vi "osa_main.vi"() -> ()   [LabVIEW 2021]
uses:
  <vilib>/Instr/_visa.llb/Select Event Type.ctl
  osa_globals.vi
  <vilib>/Instr/_visa.llb/VISA Configure Serial Port (Instr).vi
  <vilib>/ErrorRing/Error Ring.xnode
panel:
  in  "apply changes":bool
  in  "OSB status/sensor control":i32(listbox)
  in  "serial timeout (ms)":u32=15000
  out "busy...":bool
  out "LUT":variant
  out "data file refnum":refnum<file>
  in  "teensy port":refnum<visa-resource-name>[](array[refnum])
  out "reset result":bool[](array[boolean])
  out "test result":bool[](array[boolean])
  out "teensy mounted":bool[](array[boolean])
  out "display":T1
  out "elapsed time":string="00:00:00.000"
  out "start time":timestamp format="%<%H:%M:%S%3u>T"
  in  "sensor map settings":cluster{"OSB index":u8[], "display index":i32[]}={"OSB index"=[1, 2, 3, 4, 5, 6, 7], "display index"=[26, 22, 18, 14, 10, 6, 2]}
  in  "save data":bool
  in  "data folder":path
  out "OSA status":string
  out "measuring...":bool
  in  "precision (Hz)":dbl=0.1
  in  "HS frequency (Hz)":dbl=0.5
  in  "OS frequency (Hz)":dbl=1.0
  in  "stop measurement":bool
  in  "start measurement":bool
  in  "reset":bool
  in  "test":bool
  in  "init":bool
  in  "stop VI":bool
  in  "OSB mounted":i32[](listbox)
  # "odor sensor array: main panel"
  # "Each OSB occupies 4 pixels in width on the display screens; set the display index to be which pixel you want the mid-point of the OSB short edge to be located within; no need to touch this unless doing free POGO-pin mounting"
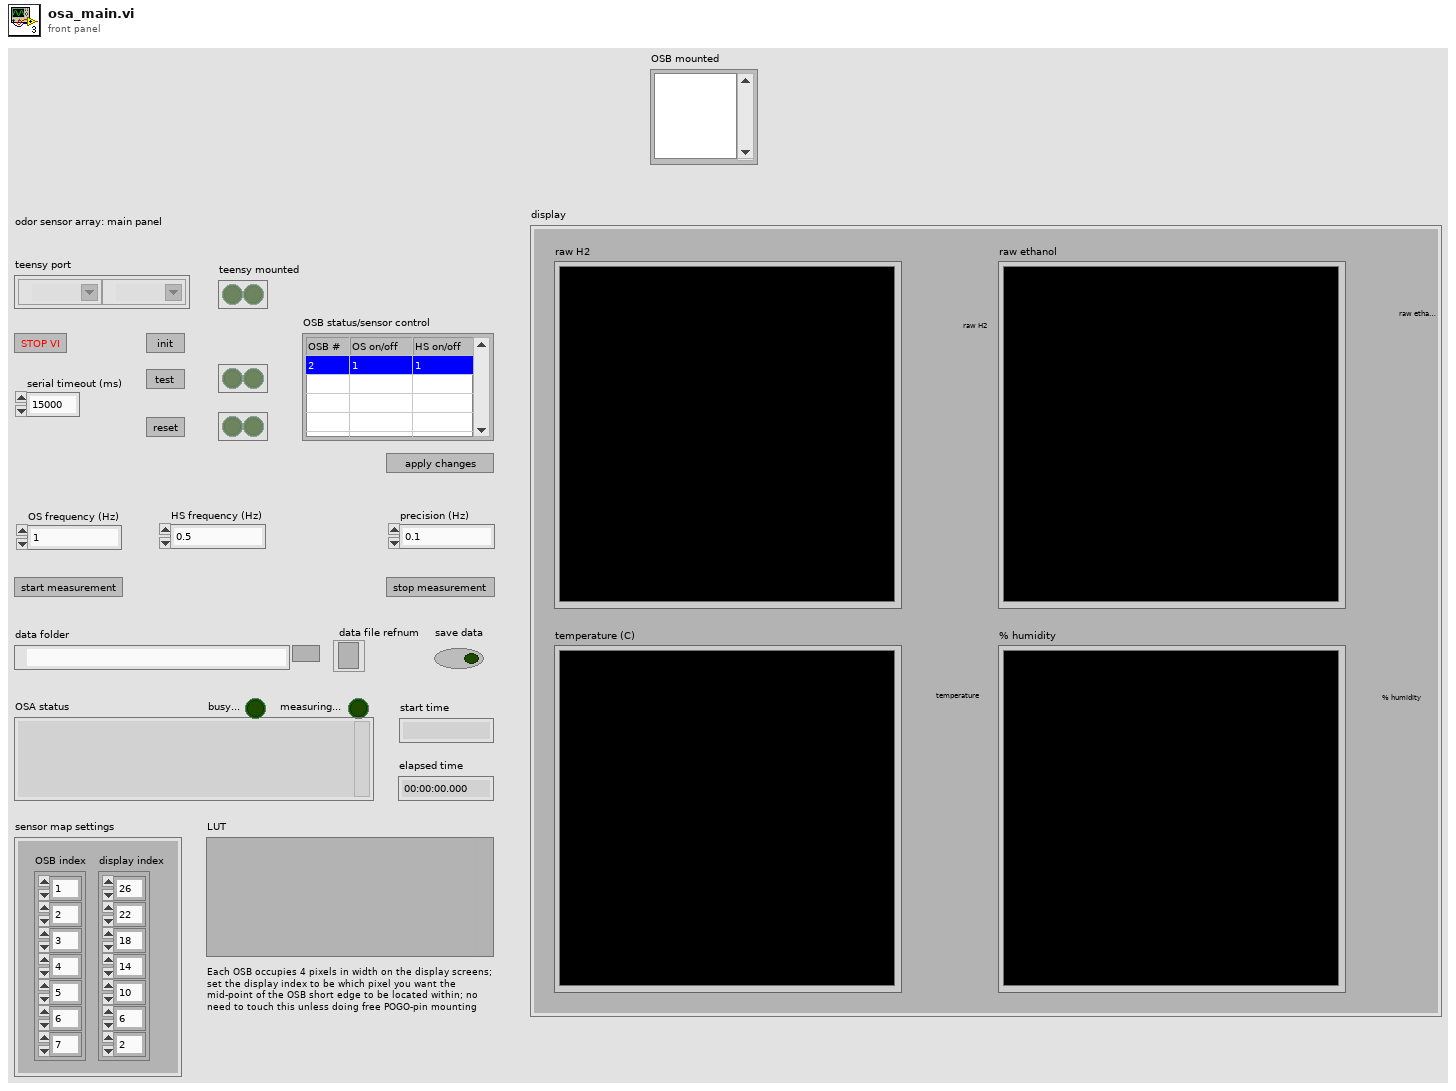
[diagram p1: front panel]
types:
  T1 = cluster{"raw ethanol":dbl[][], "raw H2":dbl[][], "temperature (C)":dbl[][], "% humidity":dbl[][]}
  T2 = cluster{"raw H2":refnum<vi>, "raw ethanol":refnum<vi>, "temperature (C)":refnum<vi>, "% humidity":refnum<vi>}
  T3 = typedef "Select Event Type.ctl" = u32
  T4 = enum16{"big-endian, network order", "native, host order", "little-endian"}
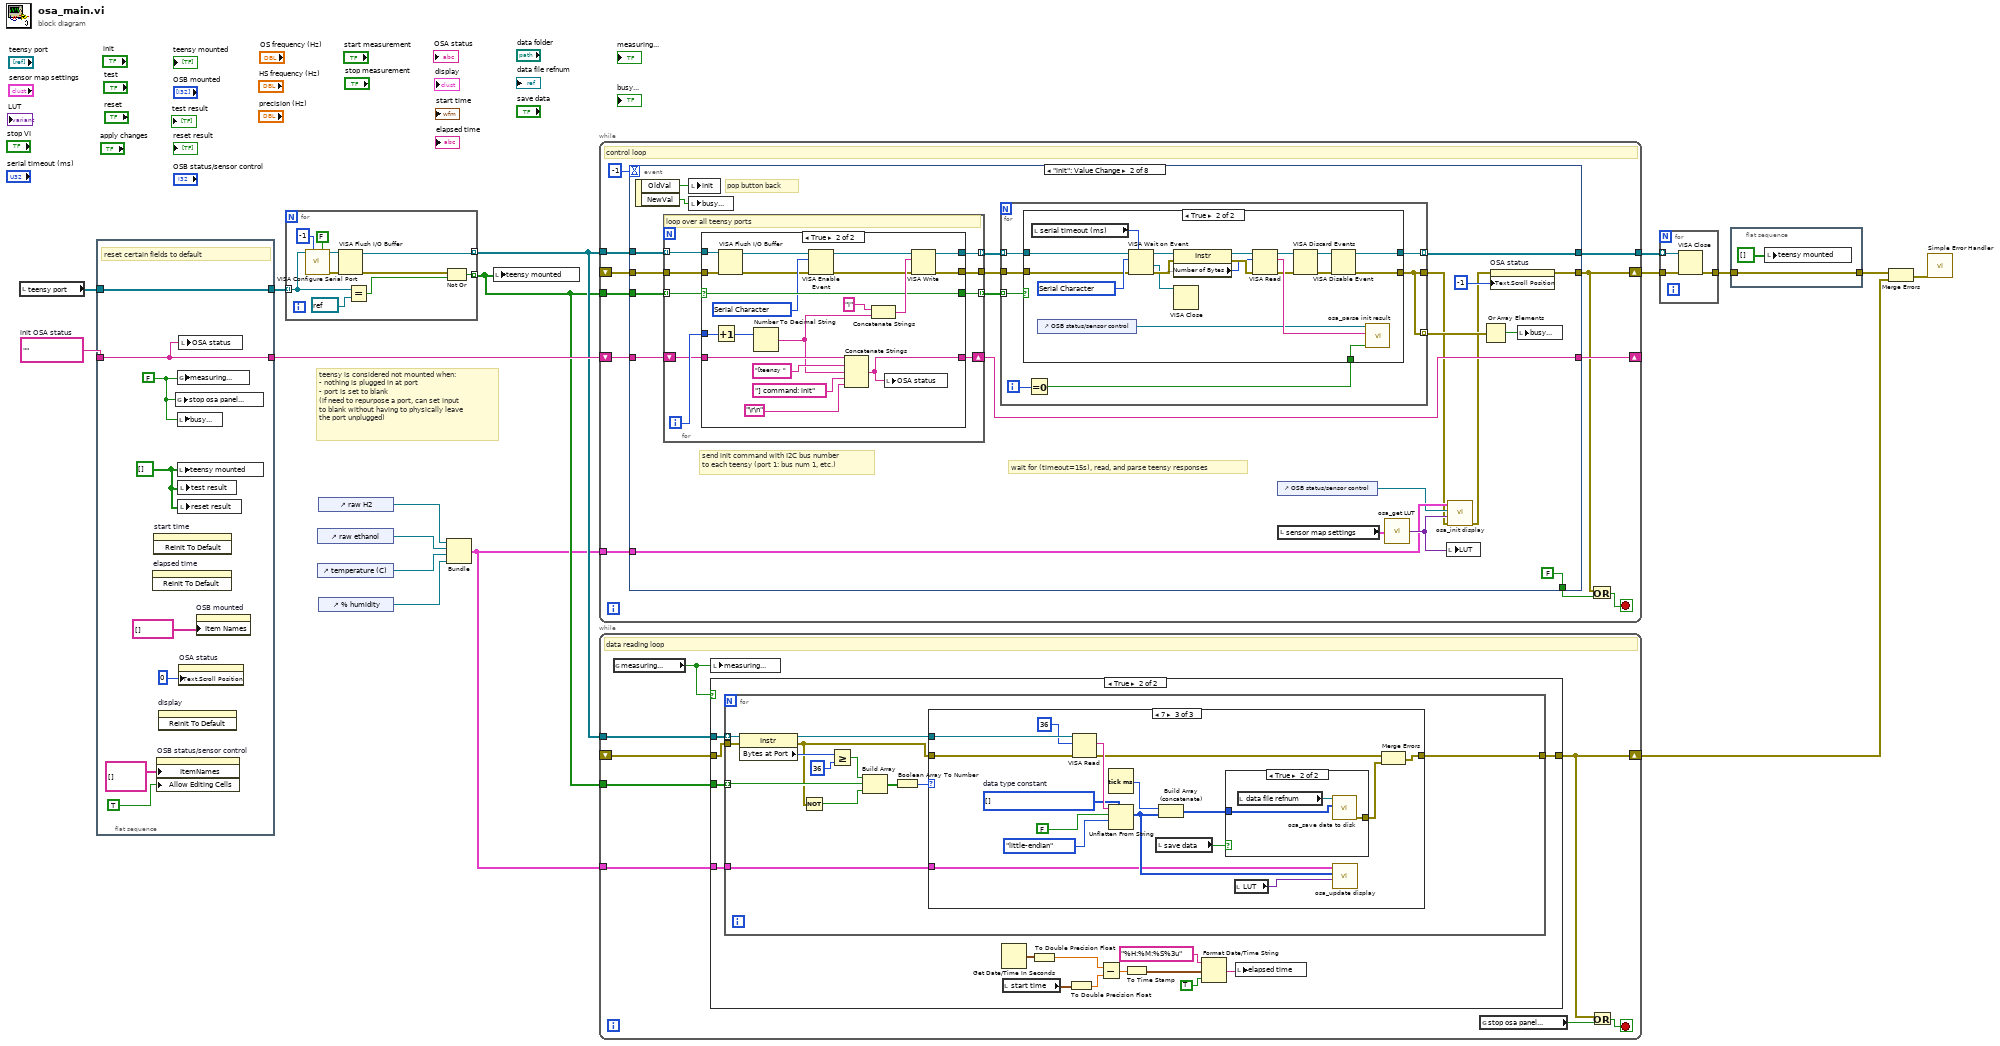
[diagram p0: block diagram]
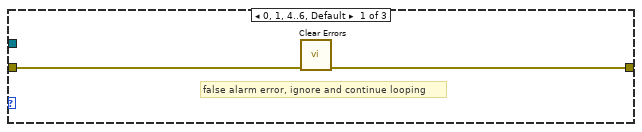
[diagram p3: hidden frame]
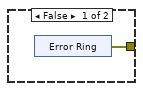
[diagram p5: hidden frame]
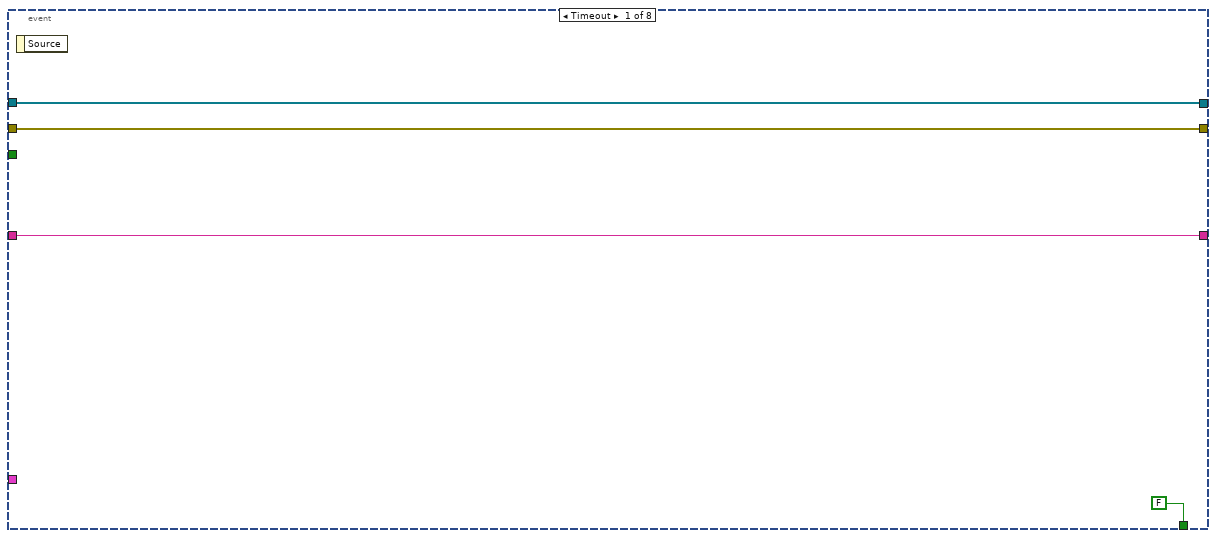
[diagram p6: hidden frame]
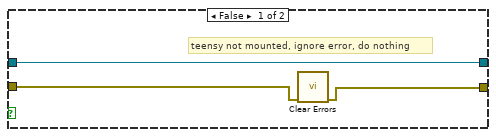
[diagram p7: hidden frame]
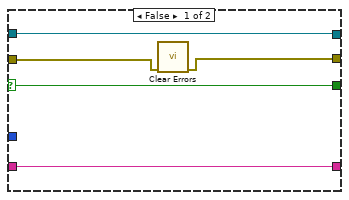
[diagram p8: hidden frame]
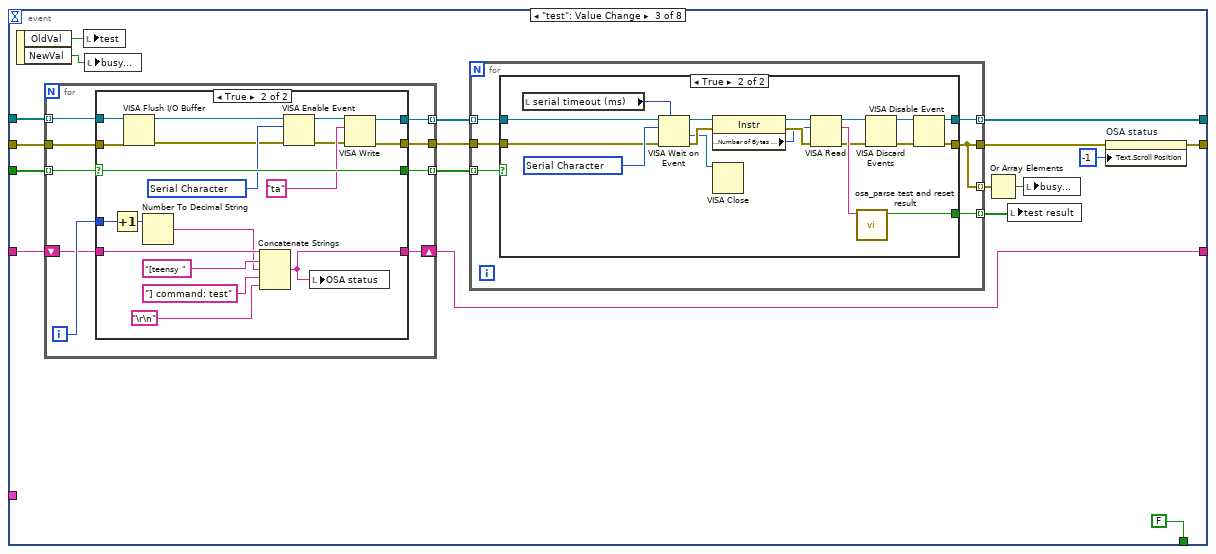
[diagram p9: hidden frame]
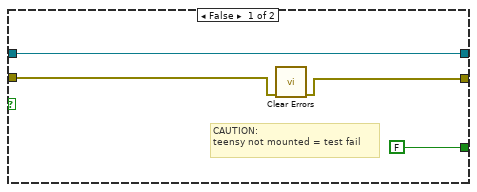
[diagram p10: hidden frame]
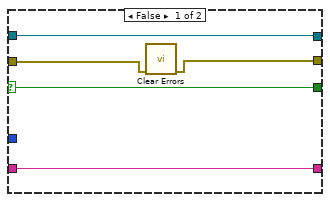
[diagram p11: hidden frame]
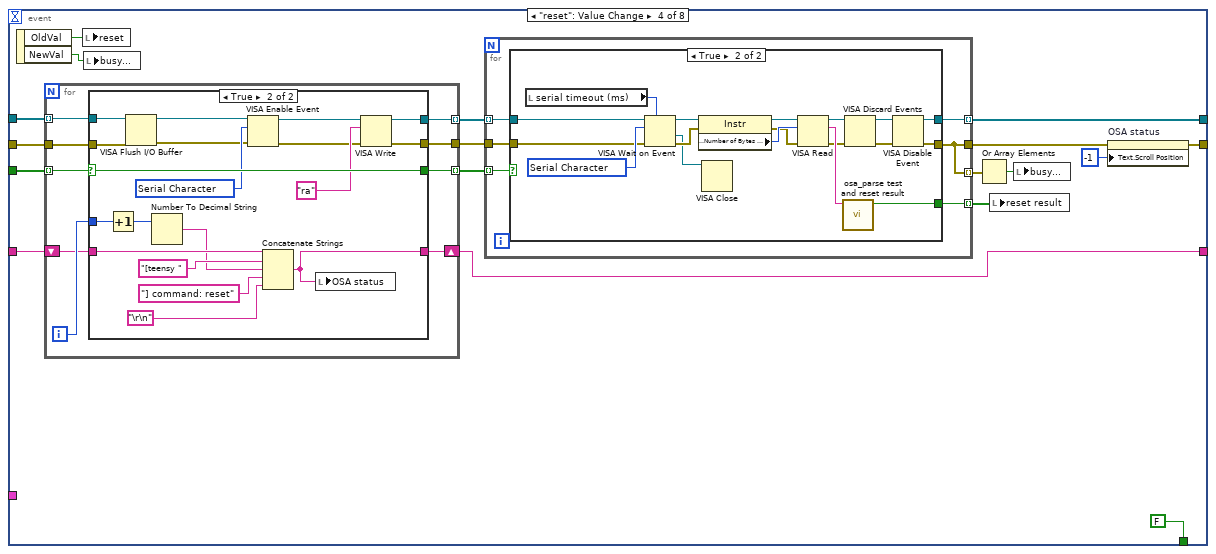
[diagram p12: hidden frame]
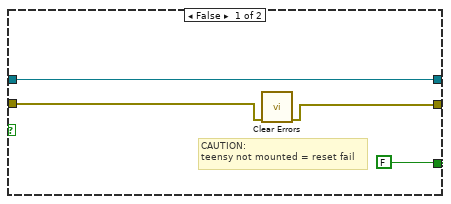
[diagram p13: hidden frame]
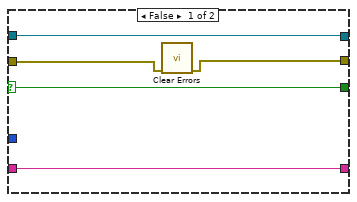
[diagram p14: hidden frame]
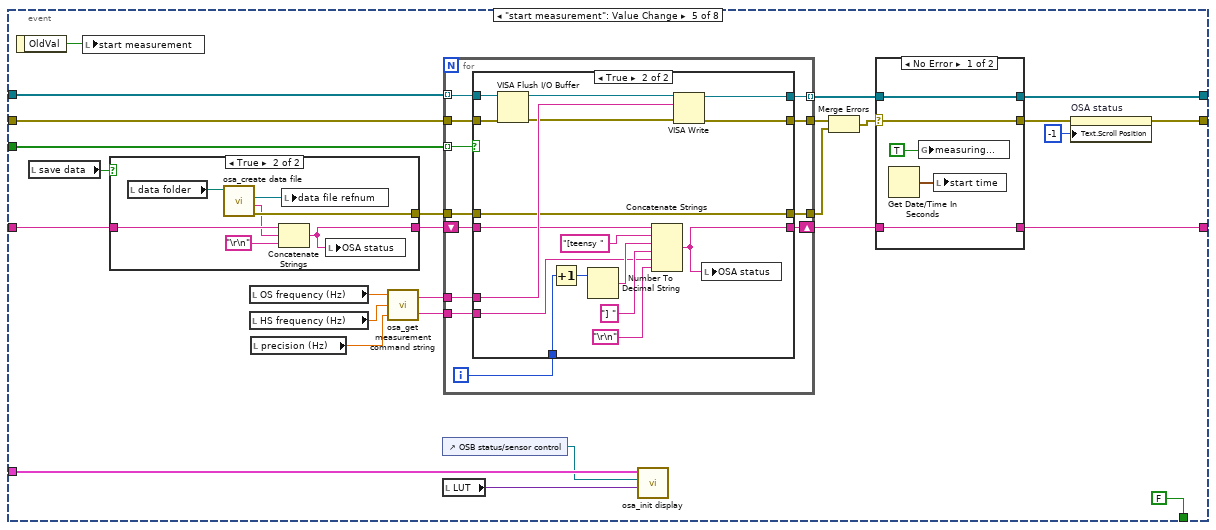
[diagram p15: hidden frame]
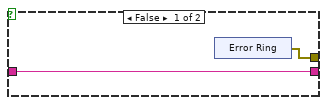
[diagram p17: hidden frame]
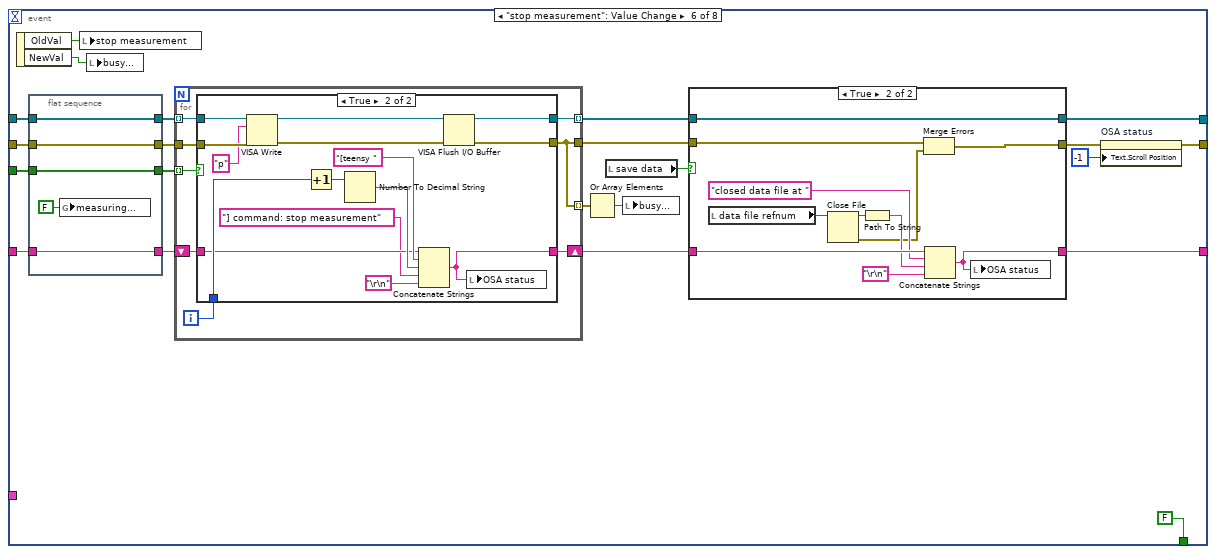
[diagram p19: hidden frame]
diagram:
  w17 = ""  # init OSA status
  # "teensy is considered not mounted when:\n- nothing is plugged in at port\n- port is set to blank\n(if need to repurpose a port, can set input\nto blank without having to physically leave\nthe port unplugged)"
  n1 = local read "teensy port"() -> (w15:refnum<visa-resource-name>[])
  n2 = flat-sequence {
    tunnel: w17 -> [w23]
    tunnel: [w23] -> w16
    tunnel: [w21] -> w14
    tunnel: w15 -> [w21]
    frame #0 {
      w22 = bool[] []
      w20 = FALSE
      # "reset certain fields to default"
      n3 = invoke on="elapsed time" class="Str" method="Reinit To Default"() -> ()  [unwired: 3 in, 3 out]
      n4 = invoke on="start time" class="AbsTime (strict)" method="Reinit To Default"() -> ()  [unwired: 3 in, 3 out]
      n5 = property on="OSB status/sensor control" class="MCListbox (strict)"("ItemNames"=string[][] [] ("Item Names"), "Allow Editing Cells"=TRUE) -> ()  [unwired: 2 in, 2 out]
      n6 = invoke on="display" class="Clust (strict)" method="Reinit To Default"() -> ()  [unwired: 3 in, 3 out]
      n7 = global write "osa_globals.vi" "stop osa panel..."(w20) -> ()
      n8 = global write "osa_globals.vi" "measuring..."(w20) -> ()
      n9 = local write "busy..."(w20) -> ()
      n10 = local write "teensy mounted"(w22) -> ()
      n11 = local write "test result"(w22) -> ()
      n12 = local write "reset result"(w22) -> ()
      n13 = local write "OSA status"(w23) -> ()
      n14 = property on="OSA status" class="Str"("Text.Scroll Position"=u32 0) -> ()  [unwired: 2 in, 2 out]
      n15 = property on="OSB mounted" class="LstBox (strict)"("Item Names"=string[] []) -> ()  [unwired: 2 in, 2 out]
    }
  }
  n16 = for {
    tunnel: w14 -> [w33] mode=indexing
    tunnel: [w30] -> w12 mode=indexing
    tunnel: [w27] -> w13 mode=indexing
    n17 = call-poly "VISA Configure Serial Port"("VISA resource name"=w33, "timeout (10sec)"=-1, "Enable Termination\nChar (T)"=FALSE) -> ("VISA resource name out"=w28:refnum<visa-resource-name>, "error out"=w29:errorcluster)  [unwired: 11 in]
    n18 = VISA Flush I/O Buffer(VISA resource name=w28, error in (no error)=w29) -> (VISA resource name out=w27:refnum<visa-resource-name>, error out=w26:errorcluster)  [unwired: 1 in]
    n19 = Equal?(x=w33, y=refnum<visa-resource-name> refnum ("teensy port 1")) -> (x = y?=w31:bool)
    n20 = Not Or(1:w31, 2:w26) -> (0:w30:bool)
  }
  n21 = control-ref of="raw ethanol"() -> (w10:refnum<vi>)
  n22 = control-ref of="temperature (C)"() -> (w9:refnum<vi>)
  n23 = control-ref of="raw H2"() -> (w11:refnum<vi>)
  n24 = control-ref of="% humidity"() -> (w8:refnum<vi>)
  n25 = Bundle("raw H2"=w11, "raw ethanol"=w10, "temperature (C)"=w9, "% humidity"=w8) -> (w7:T2)  [unwired: 1 in]
  n26 = local write "teensy mounted"(w12) -> ()
  n27 = while {
    shift-right: [w42] -> _
    shift-left: w16 -> [w44]
    tunnel: w13 -> [w45]
    tunnel: w12 -> [w43]
    shift-right: [w37] -> w5
    shift-left: _ -> [w41]
    tunnel: [w40] -> w6
    tunnel: w7 -> [w39]
    stop <- w38 stop-if-true
    # "control loop"
    n28 = event shown="[1] \"init\": Value Change" {
      selector: _ -> [_ _ _ _ _ _ _ _]
      dyn-events: _ -> [_ _ _ _ _ _ _ _]
      timeout: -1 -> [_ _ _ _ _ _ _ _]
      tunnel: w45 -> [w49 w71 w152 w231 w319 w392 w466 w562]
      tunnel: w44 -> [w47 w69 w150 w229 w311 w386 w448 w563]
      tunnel: w43 -> [_ w70 w151 w230 w318 w388 w464 _]
      tunnel: [w47 w65 w148 w227 w302 w381 w446 w563] -> w42
      tunnel: [w48 w55 w138 w218 w296 w373 w449 w564] -> w37
      tunnel: w41 -> [w48 w63 w149 w228 w298 w390 w465 w564]
      tunnel: [w49 w64 w143 w221 w304 w380 w450 w562] -> w40
      tunnel: w39 -> [_ w60 _ _ w300 _ w442 _]
      tunnel: [FALSE FALSE FALSE FALSE FALSE FALSE FALSE TRUE] -> w36
      event Timeout {
        n29 = event-data() -> ()  [unwired: 1 in, 1 out]
      }
      event "init": Value Change {
        # "wait for (timeout=15s), read, and parse teensy responses"
        # "send init command with I2C bus number\nto each teensy (port 1: bus num 1, etc.)"
        # "pop button back"
        n30 = event-data() -> ("OldVal"=w72:bool, "NewVal"=w58:bool)  [unwired: 1 in]
        n31 = for {
          tunnel: w71 -> [w109] mode=indexing
          tunnel: w70 -> [w110] mode=indexing
          tunnel: [w107] -> w68 mode=indexing
          tunnel: [w106] -> w67
          shift-right: [w104] -> w65
          shift-left: w69 -> [w105]
          tunnel: [w103] -> w66 mode=indexing
          tunnel: w63 -> [w102]
          i -> [w108]
          # "loop over all teensy ports"
          n32 = case shown="True" w110 {
            selector: w110 -> [w114 w131]
            tunnel: w109 -> [w115 w122]
            tunnel: w108 -> [_ w125]
            tunnel: [w115 w134] -> w107
            tunnel: [w111 w133] -> w106
            tunnel: [w114 w131] -> w103
            tunnel: w105 -> [w113 w130]
            tunnel: [w113 w123] -> w104
            tunnel: w102 -> [w112 w121]
            frame False {
              n33 = call <vilib>:"Clear Errors.vi"("error in (no error)"=w112) -> ("error out"=w111:errorcluster)  [unwired: 5 in, 1 out]
            }
            frame True {
              w119 = T3 1073684533 items=["Service Request"=1073684491, "Trigger"=3221168138, "Clear"=1073684493, "VXI Signal"=1073684512, "VXI/VME Interrupt"=3221168161, "VXI/VME Sysfail"=1073684509, "VXI/VME Sysreset"=1073684510, "GPIB CIC"=1073684498, "GPIB Talk"=1073684499, "GPIB Listen"=1073684500, "PXI Interrupt"=1073684514, "Serial Break"=1073684515, "Serial TermChar"=1073684516, "Serial CTS"=1073684521, "Serial DSR"=1073684522, "Serial DCD"=1073684524, "Serial RI"=1073684526, "Serial Character"=1073684533, "USB Interrupt"=1073684535, "All Enabled"=1073709055] ("Event Type")
              n34 = Increment(x=w125) -> (x+1=w124:i32)
              n35 = VISA Flush I/O Buffer(VISA resource name=w122, error in (no error)=w121) -> (VISA resource name out=w120:refnum<visa-resource-name>, error out=w118:errorcluster)  [unwired: 1 in]
              n36 = Number To Decimal String(number=w124) -> (decimal integer string=w128:string)  [unwired: 1 in]
              n37 = VISA Enable Event(8:w118, 10:w119, 11:w120) -> (0:w116:errorcluster, 3:w117:refnum<visa-resource-name>)  [unwired: 1 in]
              n38 = Concatenate Strings(w130, "[teensy ", w128, "] command: init", "\r\n") -> (w123:string)
              n39 = Concatenate Strings("i", w128) -> (w132:string)
              n40 = local write "OSA status"(w123) -> ()
              n41 = VISA Write(VISA resource name=w117, write buffer=w132, error in (no error)=w116) -> (VISA resource name out=w134:refnum<visa-resource-name>, error out=w133:errorcluster)  [unwired: 1 out]
            }
          }
        }
        n42 = local write "init"(w72) -> ()
        n43 = local write "busy..."(w58) -> ()
        n44 = for {
          tunnel: w68 -> [w78] mode=indexing
          tunnel: w67 -> [w76]
          tunnel: w66 -> [w79] mode=indexing
          tunnel: [w77] -> w64 mode=indexing
          tunnel: [w74] -> w52
          tunnel: [w74] -> w57 mode=indexing
          i -> [w75]
          n45 = Equal To 0?(x=w75) -> (x = 0?=w73:bool)
          n46 = case shown="True" w79 {
            tunnel: [w82 w85] -> w77
            tunnel: w78 -> [w82 w100]
            tunnel: w76 -> [w81 w99]
            tunnel: [w80 w84] -> w74
            tunnel: w73 -> [_ w90]
            frame False {
              # "teensy not mounted, ignore error, do nothing"
              n47 = call <vilib>:"Clear Errors.vi"("error in (no error)"=w81) -> ("error out"=w80:errorcluster)  [unwired: 5 in, 1 out]
            }
            frame True {
              w101 = T3 1073684533 items=["Service Request"=1073684491, "Trigger"=3221168138, "Clear"=1073684493, "VXI Signal"=1073684512, "VXI/VME Interrupt"=3221168161, "VXI/VME Sysfail"=1073684509, "VXI/VME Sysreset"=1073684510, "GPIB CIC"=1073684498, "GPIB Talk"=1073684499, "GPIB Listen"=1073684500, "PXI Interrupt"=1073684514, "Serial Break"=1073684515, "Serial TermChar"=1073684516, "Serial CTS"=1073684521, "Serial DSR"=1073684522, "Serial DCD"=1073684524, "Serial RI"=1073684526, "Serial Character"=1073684533, "USB Interrupt"=1073684535, "All Enabled"=1073709055] ("Event Type")
              n48 = local read "serial timeout (ms)"() -> (w91:u32)
              n49 = control-ref of="OSB status/sensor control"() -> (w83:refnum<vi>)
              n50 = VISA Wait on Event(7:w91, 8:w99, 10:w101, 11:w100) -> (0:w97:errorcluster, 1:w96:refnum<visa-resource-name>, 3:w98:refnum<visa-resource-name>)  [unwired: 1 in, 1 out]
              n51 = property class="Instr"(reference=w98, error in=w97) -> (reference out=w95:refnum<visa-resource-name>, error out=w94:errorcluster, "Serial Settings:Number of Bytes at Serial Port"=w93:u32)
              n52 = VISA Close(VISA resource name=w96) -> ()  [unwired: 1 in, 1 out]
              n53 = VISA Read(VISA resource name=w95, byte count=w93, error in (no error)=w94) -> (VISA resource name out=w88:refnum<visa-resource-name>, read buffer=w92:string, error out=w89:errorcluster)  [unwired: 1 out]
              n54 = VISA Discard Events(8:w89, 11:w88) -> (0:w87:errorcluster, 3:w86:refnum<visa-resource-name>)  [unwired: 2 in]
              n55 = VISA Disable Event(8:w87, 11:w86) -> (0:w84:errorcluster, 3:w85:refnum<visa-resource-name>)  [unwired: 2 in]
              n56 = call "osa_parse init result.vi"("wipe content?"=w90, "serial response in"=w92, "OSB status/control refnum in"=w83) -> ()  [unwired: 9 in]
            }
          }
        }
        n57 = control-ref of="OSB status/sensor control"() -> (w53:refnum<vi>)
        n58 = local read "sensor map settings"() -> (w62:cluster{"OSB index":u8[], "display index":i32[]})
        n59 = call "osa_get LUT.vi"("sensor map settings"=w62) -> ("sensor LUT"=w61:variant)  [unwired: 6 in]
        n60 = local write "LUT"(w61) -> ()
        n61 = call "osa_init display.vi"("error in (no error)"=w52, "sensor LUT"=w61, "OSB status/control refnum in"=w53, "display refnums in"=w60) -> ("error out"=w51:errorcluster)  [unwired: 6 in, 1 out]
        n62 = Or Array Elements(Boolean array=w57) -> (logical OR=w56:bool)
        n63 = property on="OSA status" class="Str"(error in=w51, "Text.Scroll Position"=-1) -> (error out=w55:errorcluster)  [unwired: 1 in, 1 out]
        n64 = local write "busy..."(w56) -> ()
      }
      event "test": Value Change {
        n65 = event-data() -> ("OldVal"=w153:bool, "NewVal"=w142:bool)  [unwired: 1 in]
        n66 = for {
          tunnel: w152 -> [w189] mode=indexing
          tunnel: w151 -> [w190] mode=indexing
          tunnel: [w187] -> w146 mode=indexing
          tunnel: [w186] -> w145
          shift-right: [w184] -> w148
          shift-left: w150 -> [w185]
          tunnel: [w183] -> w144 mode=indexing
          tunnel: w149 -> [w182]
          i -> [w188]
          n67 = case shown="True" w190 {
            selector: w190 -> [w194 w212]
            tunnel: w189 -> [w195 w202]
            tunnel: w188 -> [_ w205]
            tunnel: [w195 w214] -> w187
            tunnel: [w191 w213] -> w186
            tunnel: [w194 w212] -> w183
            tunnel: w185 -> [w193 w211]
            tunnel: [w193 w203] -> w184
            tunnel: w182 -> [w192 w201]
            frame False {
              n68 = call <vilib>:"Clear Errors.vi"("error in (no error)"=w192) -> ("error out"=w191:errorcluster)  [unwired: 5 in, 1 out]
            }
            frame True {
              w199 = T3 1073684533 items=["Service Request"=1073684491, "Trigger"=3221168138, "Clear"=1073684493, "VXI Signal"=1073684512, "VXI/VME Interrupt"=3221168161, "VXI/VME Sysfail"=1073684509, "VXI/VME Sysreset"=1073684510, "GPIB CIC"=1073684498, "GPIB Talk"=1073684499, "GPIB Listen"=1073684500, "PXI Interrupt"=1073684514, "Serial Break"=1073684515, "Serial TermChar"=1073684516, "Serial CTS"=1073684521, "Serial DSR"=1073684522, "Serial DCD"=1073684524, "Serial RI"=1073684526, "Serial Character"=1073684533, "USB Interrupt"=1073684535, "All Enabled"=1073709055] ("Event Type")
              n69 = Increment(x=w205) -> (x+1=w204:i32)
              n70 = VISA Flush I/O Buffer(VISA resource name=w202, error in (no error)=w201) -> (VISA resource name out=w200:refnum<visa-resource-name>, error out=w198:errorcluster)  [unwired: 1 in]
              n71 = Number To Decimal String(number=w204) -> (decimal integer string=w209:string)  [unwired: 1 in]
              n72 = Concatenate Strings(w211, "[teensy ", w209, "] command: test", "\r\n") -> (w203:string)
              n73 = VISA Enable Event(8:w198, 10:w199, 11:w200) -> (0:w196:errorcluster, 3:w197:refnum<visa-resource-name>)  [unwired: 1 in]
              n74 = local write "OSA status"(w203) -> ()
              n75 = VISA Write(VISA resource name=w197, write buffer="ta", error in (no error)=w196) -> (VISA resource name out=w214:refnum<visa-resource-name>, error out=w213:errorcluster)  [unwired: 1 out]
            }
          }
        }
        n76 = local write "test"(w153) -> ()
        n77 = local write "busy..."(w142) -> ()
        n78 = for {
          tunnel: w146 -> [w158] mode=indexing
          tunnel: w145 -> [w157]
          tunnel: w144 -> [w159] mode=indexing
          tunnel: [w156] -> w143 mode=indexing
          tunnel: [w155] -> w136
          tunnel: [w155] -> w140 mode=indexing
          tunnel: [w154] -> w139 mode=indexing
          n79 = case shown="True" w159 {
            tunnel: w158 -> [w163 w180]
            tunnel: w157 -> [w162 w178]
            tunnel: [w163 w165] -> w156
            tunnel: [w161 w164] -> w155
            tunnel: [FALSE w170] -> w154
            frame False {
              # "CAUTION:\nteensy not mounted = test fail"
              n80 = call <vilib>:"Clear Errors.vi"("error in (no error)"=w162) -> ("error out"=w161:errorcluster)  [unwired: 5 in, 1 out]
            }
            frame True {
              w181 = T3 1073684533 items=["Service Request"=1073684491, "Trigger"=3221168138, "Clear"=1073684493, "VXI Signal"=1073684512, "VXI/VME Interrupt"=3221168161, "VXI/VME Sysfail"=1073684509, "VXI/VME Sysreset"=1073684510, "GPIB CIC"=1073684498, "GPIB Talk"=1073684499, "GPIB Listen"=1073684500, "PXI Interrupt"=1073684514, "Serial Break"=1073684515, "Serial TermChar"=1073684516, "Serial CTS"=1073684521, "Serial DSR"=1073684522, "Serial DCD"=1073684524, "Serial RI"=1073684526, "Serial Character"=1073684533, "USB Interrupt"=1073684535, "All Enabled"=1073709055] ("Event Type")
              n81 = local read "serial timeout (ms)"() -> (w179:u32)
              n82 = VISA Wait on Event(7:w179, 8:w178, 10:w181, 11:w180) -> (0:w176:errorcluster, 1:w175:refnum<visa-resource-name>, 3:w177:refnum<visa-resource-name>)  [unwired: 1 in, 1 out]
              n83 = property class="Instr"(reference=w177, error in=w176) -> (reference out=w174:refnum<visa-resource-name>, error out=w173:errorcluster, "Serial Settings:Number of Bytes at Serial Port"=w172:u32)
              n84 = VISA Close(VISA resource name=w175) -> ()  [unwired: 1 in, 1 out]
              n85 = VISA Read(VISA resource name=w174, byte count=w172, error in (no error)=w173) -> (VISA resource name out=w168:refnum<visa-resource-name>, read buffer=w171:string, error out=w169:errorcluster)  [unwired: 1 out]
              n86 = call "osa_parse test and reset result.vi"("serial response in"=w171) -> ("test/reset result"=w170:bool)  [unwired: 9 in, 1 out]
              n87 = VISA Discard Events(8:w169, 11:w168) -> (0:w167:errorcluster, 3:w166:refnum<visa-resource-name>)  [unwired: 2 in]
              n88 = VISA Disable Event(8:w167, 11:w166) -> (0:w164:errorcluster, 3:w165:refnum<visa-resource-name>)  [unwired: 2 in]
            }
          }
        }
        n89 = Or Array Elements(Boolean array=w140) -> (logical OR=w141:bool)
        n90 = local write "test result"(w139) -> ()
        n91 = local write "busy..."(w141) -> ()
        n92 = property on="OSA status" class="Str"(error in=w136, "Text.Scroll Position"=-1) -> (error out=w138:errorcluster)  [unwired: 1 in, 1 out]
      }
      event "reset": Value Change {
        n93 = event-data() -> ("OldVal"=w232:bool, "NewVal"=w225:bool)  [unwired: 1 in]
        n94 = for {
          tunnel: w231 -> [w268] mode=indexing
          tunnel: w230 -> [w269] mode=indexing
          tunnel: [w266] -> w224 mode=indexing
          tunnel: [w265] -> w223
          shift-right: [w263] -> w227
          shift-left: w229 -> [w264]
          tunnel: [w262] -> w222 mode=indexing
          tunnel: w228 -> [w261]
          i -> [w267]
          n95 = case shown="True" w269 {
            selector: w269 -> [w273 w291]
            tunnel: w268 -> [w274 w281]
            tunnel: w267 -> [_ w284]
            tunnel: [w274 w293] -> w266
            tunnel: [w270 w292] -> w265
            tunnel: [w273 w291] -> w262
            tunnel: w264 -> [w272 w290]
            tunnel: [w272 w282] -> w263
            tunnel: w261 -> [w271 w280]
            frame False {
              n96 = call <vilib>:"Clear Errors.vi"("error in (no error)"=w271) -> ("error out"=w270:errorcluster)  [unwired: 5 in, 1 out]
            }
            frame True {
              w279 = T3 1073684533 items=["Service Request"=1073684491, "Trigger"=3221168138, "Clear"=1073684493, "VXI Signal"=1073684512, "VXI/VME Interrupt"=3221168161, "VXI/VME Sysfail"=1073684509, "VXI/VME Sysreset"=1073684510, "GPIB CIC"=1073684498, "GPIB Talk"=1073684499, "GPIB Listen"=1073684500, "PXI Interrupt"=1073684514, "Serial Break"=1073684515, "Serial TermChar"=1073684516, "Serial CTS"=1073684521, "Serial DSR"=1073684522, "Serial DCD"=1073684524, "Serial RI"=1073684526, "Serial Character"=1073684533, "USB Interrupt"=1073684535, "All Enabled"=1073709055] ("Event Type")
              n97 = Increment(x=w284) -> (x+1=w283:i32)
              n98 = VISA Flush I/O Buffer(VISA resource name=w281, error in (no error)=w280) -> (VISA resource name out=w278:refnum<visa-resource-name>, error out=w277:errorcluster)  [unwired: 1 in]
              n99 = Number To Decimal String(number=w283) -> (decimal integer string=w288:string)  [unwired: 1 in]
              n100 = VISA Enable Event(8:w277, 10:w279, 11:w278) -> (0:w275:errorcluster, 3:w276:refnum<visa-resource-name>)  [unwired: 1 in]
              n101 = Concatenate Strings(w290, "[teensy ", w288, "] command: reset", "\r\n") -> (w282:string)
              n102 = local write "OSA status"(w282) -> ()
              n103 = VISA Write(VISA resource name=w276, write buffer="ra", error in (no error)=w275) -> (VISA resource name out=w293:refnum<visa-resource-name>, error out=w292:errorcluster)  [unwired: 1 out]
            }
          }
        }
        n104 = local write "reset"(w232) -> ()
        n105 = local write "busy..."(w225) -> ()
        n106 = for {
          tunnel: w224 -> [w237] mode=indexing
          tunnel: w223 -> [w235]
          tunnel: w222 -> [w238] mode=indexing
          tunnel: [w236] -> w221 mode=indexing
          tunnel: [w234] -> w217
          tunnel: [w234] -> w216 mode=indexing
          tunnel: [w233] -> w219 mode=indexing
          n107 = case shown="True" w238 {
            tunnel: [w242 w244] -> w236
            tunnel: w237 -> [w242 w260]
            tunnel: w235 -> [w241 w257]
            tunnel: [w240 w243] -> w234
            tunnel: [FALSE w249] -> w233
            frame False {
              # "CAUTION:\nteensy not mounted = reset fail"
              n108 = call <vilib>:"Clear Errors.vi"("error in (no error)"=w241) -> ("error out"=w240:errorcluster)  [unwired: 5 in, 1 out]
            }
            frame True {
              w258 = T3 1073684533 items=["Service Request"=1073684491, "Trigger"=3221168138, "Clear"=1073684493, "VXI Signal"=1073684512, "VXI/VME Interrupt"=3221168161, "VXI/VME Sysfail"=1073684509, "VXI/VME Sysreset"=1073684510, "GPIB CIC"=1073684498, "GPIB Talk"=1073684499, "GPIB Listen"=1073684500, "PXI Interrupt"=1073684514, "Serial Break"=1073684515, "Serial TermChar"=1073684516, "Serial CTS"=1073684521, "Serial DSR"=1073684522, "Serial DCD"=1073684524, "Serial RI"=1073684526, "Serial Character"=1073684533, "USB Interrupt"=1073684535, "All Enabled"=1073709055] ("Event Type")
              n109 = local read "serial timeout (ms)"() -> (w259:u32)
              n110 = VISA Wait on Event(7:w259, 8:w257, 10:w258, 11:w260) -> (0:w255:errorcluster, 1:w254:refnum<visa-resource-name>, 3:w256:refnum<visa-resource-name>)  [unwired: 1 in, 1 out]
              n111 = property class="Instr"(reference=w256, error in=w255) -> (reference out=w253:refnum<visa-resource-name>, error out=w251:errorcluster, "Serial Settings:Number of Bytes at Serial Port"=w252:u32)
              n112 = VISA Close(VISA resource name=w254) -> ()  [unwired: 1 in, 1 out]
              n113 = VISA Read(VISA resource name=w253, byte count=w252, error in (no error)=w251) -> (VISA resource name out=w247:refnum<visa-resource-name>, read buffer=w250:string, error out=w248:errorcluster)  [unwired: 1 out]
              n114 = call "osa_parse test and reset result.vi"("serial response in"=w250) -> ("test/reset result"=w249:bool)  [unwired: 9 in, 1 out]
              n115 = VISA Discard Events(8:w248, 11:w247) -> (0:w246:errorcluster, 3:w245:refnum<visa-resource-name>)  [unwired: 2 in]
              n116 = VISA Disable Event(8:w246, 11:w245) -> (0:w243:errorcluster, 3:w244:refnum<visa-resource-name>)  [unwired: 2 in]
            }
          }
        }
        n117 = Or Array Elements(Boolean array=w216) -> (logical OR=w220:bool)
        n118 = local write "reset result"(w219) -> ()
        n119 = local write "busy..."(w220) -> ()
        n120 = property on="OSA status" class="Str"(error in=w217, "Text.Scroll Position"=-1) -> (error out=w218:errorcluster)  [unwired: 1 in, 1 out]
      }
      event "start measurement": Value Change {
        n121 = event-data() -> ("OldVal"=w320:bool)  [unwired: 1 in]
        n122 = local read "save data"() -> (w312:bool)
        n123 = local write "start measurement"(w320) -> ()
        n124 = case shown="True" w312 {
          tunnel: [w329 w338] -> w309
          tunnel: w311 -> [w330 w337]
          tunnel: [w330 w334] -> w310
          frame False {
            n125 = xnode "Error Ring"() -> ("error out"=w329:errorcluster)
          }
          frame True {
            n126 = local read "data folder"() -> (w333:path)
            n127 = call "osa_create data file.vi"("data folder in"=w333) -> ("error out"=w338:errorcluster, "status string"=w336:string, "data file refnum"=w332:refnum<file>)  [unwired: 7 in, 1 out]
            n128 = Concatenate Strings(w337, w336, "\r\n") -> (w334:string)
            n129 = local write "data file refnum"(w332) -> ()
            n130 = local write "OSA status"(w334) -> ()
          }
        }
        n131 = local read "OS frequency (Hz)"() -> (w315:dbl)
        n132 = local read "HS frequency (Hz)"() -> (w316:dbl)
        n133 = local read "precision (Hz)"() -> (w317:dbl)
        n134 = call "osa_get measurement command string.vi"("precision (Hz)"=w317, "HS frequency (Hz)"=w316, "OS frequency (Hz)"=w315) -> ("status string"=w313:string, "command string"=w314:string)
        n135 = control-ref of="OSB status/sensor control"() -> (w294:refnum<vi>)
        n136 = local read "LUT"() -> (w299:variant)
        n137 = for {
          tunnel: w319 -> [w350] mode=indexing
          tunnel: w298 -> [w349]
          tunnel: w318 -> [w347] mode=indexing
          tunnel: w314 -> [w348]
          tunnel: w313 -> [w344]
          shift-right: [w343] -> w303
          shift-left: w310 -> [w346]
          tunnel: [w342] -> w305 mode=indexing
          tunnel: [w341] -> w308
          tunnel: w309 -> [w340]
          tunnel: [w339] -> w307
          i -> [w345]
          n138 = case shown="True" w347 {
            tunnel: w350 -> [w353 w358]
            tunnel: w349 -> [w354 w357]
            tunnel: w348 -> [_ w371]
            tunnel: w346 -> [w352 w365]
            tunnel: w345 -> [_ w369]
            tunnel: w344 -> [_ w364]
            tunnel: [w352 w363] -> w343
            tunnel: [w354 w361] -> w341
            tunnel: [w353 w360] -> w342
            tunnel: w340 -> [w351 w359]
            tunnel: [w351 w359] -> w339
            frame False {
            }
            frame True {
              n139 = VISA Flush I/O Buffer(VISA resource name=w358, error in (no error)=w357) -> (VISA resource name out=w356:refnum<visa-resource-name>, error out=w355:errorcluster)  [unwired: 1 in]
              n140 = Increment(x=w369) -> (x+1=w370:i32)
              n141 = Number To Decimal String(number=w370) -> (decimal integer string=w368:string)  [unwired: 1 in]
              n142 = Concatenate Strings(w365, "[teensy ", w368, "] ", w364, "\r\n") -> (w363:string)
              n143 = VISA Write(VISA resource name=w356, write buffer=w371, error in (no error)=w355) -> (VISA resource name out=w360:refnum<visa-resource-name>, error out=w361:errorcluster)  [unwired: 1 out]
              n144 = local write "OSA status"(w363) -> ()
            }
          }
        }
        n145 = call "osa_init display.vi"("sensor LUT"=w299, "OSB status/control refnum in"=w294, "display refnums in"=w300) -> ()  [unwired: 7 in, 2 out]
        n146 = Merge Errors(w308, w307) -> (w306:errorcluster)
        n147 = case shown="No Error" w306 {
          selector: w306 -> [w324 w326]
          tunnel: [w325 w327] -> w304
          tunnel: w305 -> [w325 w327]
          tunnel: [w324 w326] -> w297
          tunnel: w303 -> [w322 w328]
          tunnel: [w322 w328] -> w302
          frame No Error {
            n148 = Get Date/Time In Seconds() -> (seconds since 1Jan1904=w321:timestamp)
            n149 = global write "osa_globals.vi" "measuring..."(TRUE) -> ()
            n150 = local write "start time"(w321) -> ()
          }
          frame Error {
          }
        }
        n151 = property on="OSA status" class="Str"(error in=w297, "Text.Scroll Position"=-1) -> (error out=w296:errorcluster)  [unwired: 1 in, 1 out]
      }
      event "stop measurement": Value Change {
        n152 = event-data() -> ("OldVal"=w393:bool, "NewVal"=w378:bool)  [unwired: 1 in]
        n153 = flat-sequence {
          tunnel: w392 -> [w412]
          tunnel: [w412] -> w391
          tunnel: w390 -> [w410]
          tunnel: [w410] -> w389
          tunnel: w388 -> [w409]
          tunnel: [w409] -> w387
          tunnel: w386 -> [w408]
          tunnel: [w408] -> w385
          frame #0 {
            n154 = global write "osa_globals.vi" "measuring..."(FALSE) -> ()
          }
        }
        n155 = local write "stop measurement"(w393) -> ()
        n156 = local write "busy..."(w378) -> ()
        n157 = for {
          tunnel: w391 -> [w420] mode=indexing
          tunnel: w389 -> [w419]
          tunnel: w387 -> [w418] mode=indexing
          shift-right: [w415] -> w382
          shift-left: w385 -> [w416]
          tunnel: [w414] -> w384 mode=indexing
          tunnel: [w413] -> w383
          tunnel: [w413] -> w376 mode=indexing
          i -> [w417]
          n158 = case shown="True" w418 {
            tunnel: w420 -> [w423 w438]
            tunnel: w419 -> [w422 w437]
            tunnel: w417 -> [_ w432]
            tunnel: w416 -> [w421 w431]
            tunnel: [w421 w428] -> w415
            tunnel: [w423 w425] -> w414
            tunnel: [w422 w424] -> w413
            frame False {
            }
            frame True {
              n159 = VISA Write(VISA resource name=w438, write buffer="p", error in (no error)=w437) -> (VISA resource name out=w427:refnum<visa-resource-name>, error out=w426:errorcluster)  [unwired: 1 out]
              n160 = Increment(x=w432) -> (x+1=w434:i32)
              n161 = Number To Decimal String(number=w434) -> (decimal integer string=w435:string)  [unwired: 1 in]
              n162 = Concatenate Strings(w431, "[teensy ", w435, "] command: stop measurement", "\r\n") -> (w428:string)
              n163 = VISA Flush I/O Buffer(VISA resource name=w427, error in (no error)=w426) -> (VISA resource name out=w425:refnum<visa-resource-name>, error out=w424:errorcluster)  [unwired: 1 in]
              n164 = local write "OSA status"(w428) -> ()
            }
          }
        }
        n165 = Or Array Elements(Boolean array=w376) -> (logical OR=w375:bool)
        n166 = local read "save data"() -> (w377:bool)
        n167 = local write "busy..."(w375) -> ()
        n168 = case shown="True" w377 {
          tunnel: w384 -> [w396 w407]
          tunnel: w383 -> [w395 w399]
          tunnel: [w396 w407] -> w380
          tunnel: w382 -> [w394 w404]
          tunnel: [w394 w400] -> w381
          tunnel: [w395 w397] -> w374
          frame False {
          }
          frame True {
            n169 = local read "data file refnum"() -> (w406:refnum<file>)
            n170 = Close File(refnum=w406) -> (path=w405:path, error out=w398:errorcluster)  [unwired: 1 in]
            n171 = Path To String(path=w405) -> (string=w402:string)
            n172 = Merge Errors(w399, w398) -> (w397:errorcluster)
            n173 = Concatenate Strings(w404, "closed data file at ", w402, "\r\n") -> (w400:string)
            n174 = local write "OSA status"(w400) -> ()
          }
        }
        n175 = property on="OSA status" class="Str"(error in=w374, "Text.Scroll Position"=-1) -> (error out=w373:errorcluster)  [unwired: 1 in, 1 out]
      }
      event "apply changes": Value Change {
        # "if measuring, send measurement command again to resume"
        # "send sensor on/off commands"
        # "if measuring, send interrupt first"
        n176 = event-data() -> ("OldVal"=w468:bool)  [unwired: 1 in]
        n177 = global read "osa_globals.vi" "measuring..."() -> (w439:bool)
        n178 = local write "apply changes"(w468) -> ()
        n179 = case shown="True" w439 {
          tunnel: w466 -> [w532 w541]
          tunnel: w465 -> [w531 w540]
          tunnel: w464 -> [w530 w539]
          tunnel: [w532 w538] -> w462
          tunnel: [w531 w533] -> w461
          tunnel: [w530 w535] -> w463
          frame False {
          }
          frame True {
            n180 = for {
              tunnel: w541 -> [w547] mode=indexing
              tunnel: w540 -> [w546]
              tunnel: w539 -> [w545] mode=indexing
              tunnel: [w544] -> w538 mode=indexing
              tunnel: [w543] -> w534
              tunnel: [w543] -> w536 mode=indexing
              tunnel: [w542] -> w535 mode=indexing
              n181 = case shown="True" w545 {
                selector: w545 -> [w548 w555]
                tunnel: w547 -> [w550 w558]
                tunnel: w546 -> [w549 w557]
                tunnel: [w550 w553] -> w544
                tunnel: [w549 w551] -> w543
                tunnel: [w548 w555] -> w542
                frame False {
                }
                frame True {
                  n182 = VISA Write(VISA resource name=w558, write buffer="p", error in (no error)=w557) -> (VISA resource name out=w554:refnum<visa-resource-name>, error out=w552:errorcluster)  [unwired: 1 out]
                  n183 = VISA Flush I/O Buffer(VISA resource name=w554, error in (no error)=w552) -> (VISA resource name out=w553:refnum<visa-resource-name>, error out=w551:errorcluster)  [unwired: 1 in]
                }
              }
            }
            n184 = Or Array Elements(Boolean array=w536) -> (logical OR=w537:bool)
            n185 = call "Time Delay"("error in (no error)"=w534) -> ("error out"=w533:errorcluster)  [unwired: 10 in]
            n186 = local write "busy..."(w537) -> ()
          }
        }
        n187 = control-ref of="OSB status/sensor control"() -> (w441:refnum<vi>)
        n188 = call "osa_get sensor toggle command string.vi"("OSB status/control"=w441) -> ("status string"=w447:string, "command string 2"=w459:string[], "command string 1"=w460:string[])  [unwired: 8 in]
        n189 = for {
          tunnel: w463 -> [w506] mode=indexing
          tunnel: w462 -> [w505] mode=indexing
          tunnel: w461 -> [w504]
          tunnel: w460 -> [w503]
          tunnel: w459 -> [w502]
          tunnel: [w500] -> w444
          tunnel: [w500] -> w458 mode=indexing
          tunnel: [w499] -> w452 mode=indexing
          tunnel: [w498] -> w451 mode=indexing
          i -> [w501]
          n190 = case shown="True" w506 {
            selector: w506 -> [w507 w512]
            tunnel: w505 -> [w509 w515]
            tunnel: w504 -> [w508 w514]
            tunnel: w503 -> [_ w518]
            tunnel: w502 -> [_ w517]
            tunnel: w501 -> [_ w520]
            tunnel: [w508 w510] -> w500
            tunnel: [w509 w513] -> w499
            tunnel: [w507 w511] -> w498
            frame False {
            }
            frame True {
              n191 = Equal To 0?(x=w520) -> (x = 0?=w519:bool)
              n192 = Select(t=w518, s=w519, f=w517) -> (s? t:f=w516:string[])
              n193 = for {
                tunnel: w516 -> [w529] mode=indexing
                tunnel: w514 -> [w524]
                tunnel: w512 -> [w528]
                tunnel: [w528] -> w511
                tunnel: w515 -> [w526]
                tunnel: [w527] -> w513
                tunnel: [w521] -> w510
                n194 = VISA Flush I/O Buffer(VISA resource name=w526, error in (no error)=w524) -> (VISA resource name out=w525:refnum<visa-resource-name>, error out=w523:errorcluster)  [unwired: 1 in]
                n195 = VISA Write(VISA resource name=w525, write buffer=w529, error in (no error)=w523) -> (VISA resource name out=w527:refnum<visa-resource-name>, error out=w522:errorcluster)  [unwired: 1 out]
                n196 = call "Time Delay2"("error in (no error)"=w522) -> ("error out"=w521:errorcluster)  [unwired: 10 in]
              }
            }
          }
        }
        n197 = Concatenate Strings(w448, w447, "\r\n") -> (w446:string)
        n198 = local read "OS frequency (Hz)"() -> (w456:dbl)
        n199 = local read "HS frequency (Hz)"() -> (w455:dbl)
        n200 = local read "precision (Hz)"() -> (w454:dbl)
        n201 = local write "OSA status"(w446) -> ()
        n202 = call "osa_get measurement command string.vi"("precision (Hz)"=w454, "HS frequency (Hz)"=w455, "OS frequency (Hz)"=w456) -> ("command string"=w453:string)  [unwired: 1 out]
        n203 = local read "LUT"() -> (w440:variant)
        n204 = call "osa_init display.vi"("error in (no error)"=w444, "sensor LUT"=w440, "OSB status/control refnum in"=w441, "display refnums in"=w442) -> ("error out"=w443:errorcluster)  [unwired: 6 in, 1 out]
        n205 = Or Array Elements(Boolean array=w458) -> (logical OR=w457:bool)
        n206 = case shown="True" w439 {
          tunnel: w453 -> [_ w482]
          tunnel: w452 -> [w472 w481]
          tunnel: w443 -> [w471 w480]
          tunnel: w451 -> [_ w479]
          tunnel: [w472 w476] -> w450
          tunnel: [w470 w474] -> w449
          frame False {
            n207 = property on="OSA status" class="Str"(error in=w471, "Text.Scroll Position"=-1) -> (error out=w470:errorcluster)  [unwired: 1 in, 1 out]
          }
          frame True {
            n208 = for {
              tunnel: w482 -> [w486]
              tunnel: w481 -> [w487] mode=indexing
              tunnel: w480 -> [w485]
              tunnel: w479 -> [w488] mode=indexing
              tunnel: [w483] -> w475
              tunnel: [w484] -> w476 mode=indexing
              tunnel: [w483] -> w478 mode=indexing
              n209 = case shown="True" w488 {
                tunnel: w487 -> [w490 w494]
                tunnel: w486 -> [_ w497]
                tunnel: w485 -> [w489 w492]
                tunnel: [w490 w496] -> w484
                tunnel: [w489 w495] -> w483
                frame False {
                }
                frame True {
                  n210 = VISA Flush I/O Buffer(VISA resource name=w494, error in (no error)=w492) -> (VISA resource name out=w493:refnum<visa-resource-name>, error out=w491:errorcluster)  [unwired: 1 in]
                  n211 = VISA Write(VISA resource name=w493, write buffer=w497, error in (no error)=w491) -> (VISA resource name out=w496:refnum<visa-resource-name>, error out=w495:errorcluster)  [unwired: 1 out]
                }
              }
            }
            n212 = Or Array Elements(Boolean array=w478) -> (logical OR=w477:bool)
            n213 = property on="OSA status" class="Str"(error in=w475, "Text.Scroll Position"=-1) -> (error out=w474:errorcluster)  [unwired: 1 in, 1 out]
            n214 = local write "busy..."(w477) -> ()
          }
        }
        n215 = local write "busy..."(w457) -> ()
      }
      event "stop VI": Value Change {
        n216 = event-data() -> ("OldVal"=w565:bool)  [unwired: 1 in]
        n217 = local write "stop VI"(w565) -> ()
        n218 = global write "osa_globals.vi" "stop osa panel..."(TRUE) -> ()
        n219 = global write "osa_globals.vi" "measuring..."(FALSE) -> ()
      }
    }
    n220 = Or(x=w37, y=w36) -> (x .or. y?=w38:bool)
  }
  n221 = while {
    tunnel: w13 -> [w573]
    tunnel: w12 -> [w572]
    shift-right: [w569] -> w4
    shift-left: _ -> [w570]
    tunnel: w7 -> [w571]
    stop <- w568 stop-if-true
    # "data reading loop"
    n222 = global read "osa_globals.vi" "measuring..."() -> (w566:bool)
    n223 = case shown="True" w566 {
      tunnel: w573 -> [_ w588]
      tunnel: w572 -> [_ w587]
      tunnel: w571 -> [_ w586]
      tunnel: [w574 w575] -> w569
      tunnel: w570 -> [w574 w585]
      frame False {
      }
      frame True {
        n224 = for {
          tunnel: w588 -> [w601] mode=indexing
          tunnel: w587 -> [w595] mode=indexing
          tunnel: w586 -> [w598]
          tunnel: [w597] -> w575
          tunnel: w585 -> [w596]
          # "loop over all teensy ports"
          n225 = property class="Instr"(reference=w601, error in=w596) -> (reference out=w590:refnum<visa-resource-name>, error out=w589:errorcluster, "Bytes at Port"=w599:u32)
          n226 = Not(x=w589) -> (.not. x?=w594:bool)
          n227 = Greater Or Equal?(x=w599, y=u32 36) -> (x >= y?=w593:bool)
          n228 = Build Array(w593, w595, w594) -> (w592:bool[])
          n229 = Boolean Array To Number(Boolean array=w592) -> (number=w591:u32)
          n230 = case shown="7" w591 {
            tunnel: w590 -> [_ _ w620]
            tunnel: w589 -> [w603 w604 w619]
            tunnel: w598 -> [_ _ w605]
            tunnel: [w602 w604 w613] -> w597
            frame 0, 1, 4..6, Default {
              # "false alarm error, ignore and continue looping"
              n231 = call <vilib>:"Clear Errors.vi"("error in (no error)"=w603) -> ("error out"=w602:errorcluster)  [unwired: 5 in, 1 out]
            }
            frame 2, 3 {
              # "likely a real serial error has occured, pass it along to quit VI"
            }
            frame 7 {
              w616 = u32[] []  # data type constant
              n232 = VISA Read(VISA resource name=w620, byte count=u32 36, error in (no error)=w619) -> (read buffer=w618:string, error out=w612:errorcluster)  [unwired: 2 out]
              n233 = Tick Count (ms)() -> (millisecond timer value=w607:u32)
              n234 = Unflatten From String(type=w616, binary string=w618, data includes array or string size? (T)=FALSE, byte order (0:big-endian, network order)=T4."little-endian") -> (value=w608:u32[])  [unwired: 1 in, 2 out]
              n235 = local read "save data"() -> (w615:bool)
              n236 = Build Array (concatenate)(w607, w608) -> (w606:u32[])
              n237 = case shown="True" w615 {
                tunnel: [w621 w624] -> w611
                tunnel: w606 -> [_ w623]
                frame False {
                  n238 = xnode "Error Ring"() -> ("error out"=w621:errorcluster)
                }
                frame True {
                  n239 = local read "data file refnum"() -> (w625:refnum<file>)
                  n240 = call "osa_save data to disk.vi"("data"=w623, "data file refnum in"=w625) -> ("error out"=w624:errorcluster)  [unwired: 8 in, 1 out]
                }
              }
              n241 = local read "LUT"() -> (w614:variant)
              n242 = call "osa_update display.vi"("sensor LUT"=w614, "data"=w608, "display refnums in"=w605) -> ()  [unwired: 8 in, 1 out]
              n243 = Merge Errors(w612, w611) -> (w613:errorcluster)
            }
          }
        }
        n244 = Get Date/Time In Seconds() -> (seconds since 1Jan1904=w583:timestamp)
        n245 = local read "start time"() -> (w582:timestamp)
        n246 = To Double Precision Float(number=w583) -> (double precision float=w581:dbl)
        n247 = To Double Precision Float(number=w582) -> (double precision float=w580:dbl)
        n248 = Subtract(x=w581, y=w580) -> (x-y=w579:dbl)
        n249 = To Time Stamp(1:w579) -> (0:w578:timestamp)
        n250 = Format Date/Time String(time format string (%c)="%H:%M:%S%3u", seconds (now)=w578, UTC format=TRUE) -> (date/time string=w576:string)
        n251 = local write "elapsed time"(w576) -> ()
      }
    }
    n252 = local write "measuring..."(w566) -> ()
    n253 = global read "osa_globals.vi" "stop osa panel..."() -> (w567:bool)
    n254 = Or(x=w569, y=w567) -> (x .or. y?=w568:bool)
  }
  n255 = for {
    tunnel: w6 -> [w627] mode=indexing
    tunnel: w5 -> [w628]
    tunnel: [w626] -> w2
    n256 = VISA Close(VISA resource name=w627, error in (no error)=w628) -> (error out=w626:errorcluster)
  }
  n257 = flat-sequence {
    tunnel: [w629] -> w1
    tunnel: w2 -> [w629]
    frame #0 {
      n258 = local write "teensy mounted"(bool[] []) -> ()
    }
  }
  n259 = Merge Errors(w1, w4) -> (w3:errorcluster)
  n260 = call <vilib>:"Simple Error Handler.vi"("error in (no error)"=w3) -> ()  [unwired: 4 in, 5 out]
